vi "L12_1.1.vi"() -> ()   [LabVIEW 2012]
panel:
  out "sum":i64
  out "max index(es)":i32
  out "max value":dbl
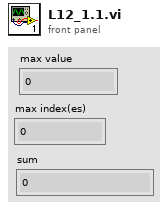
[diagram p1: front panel]
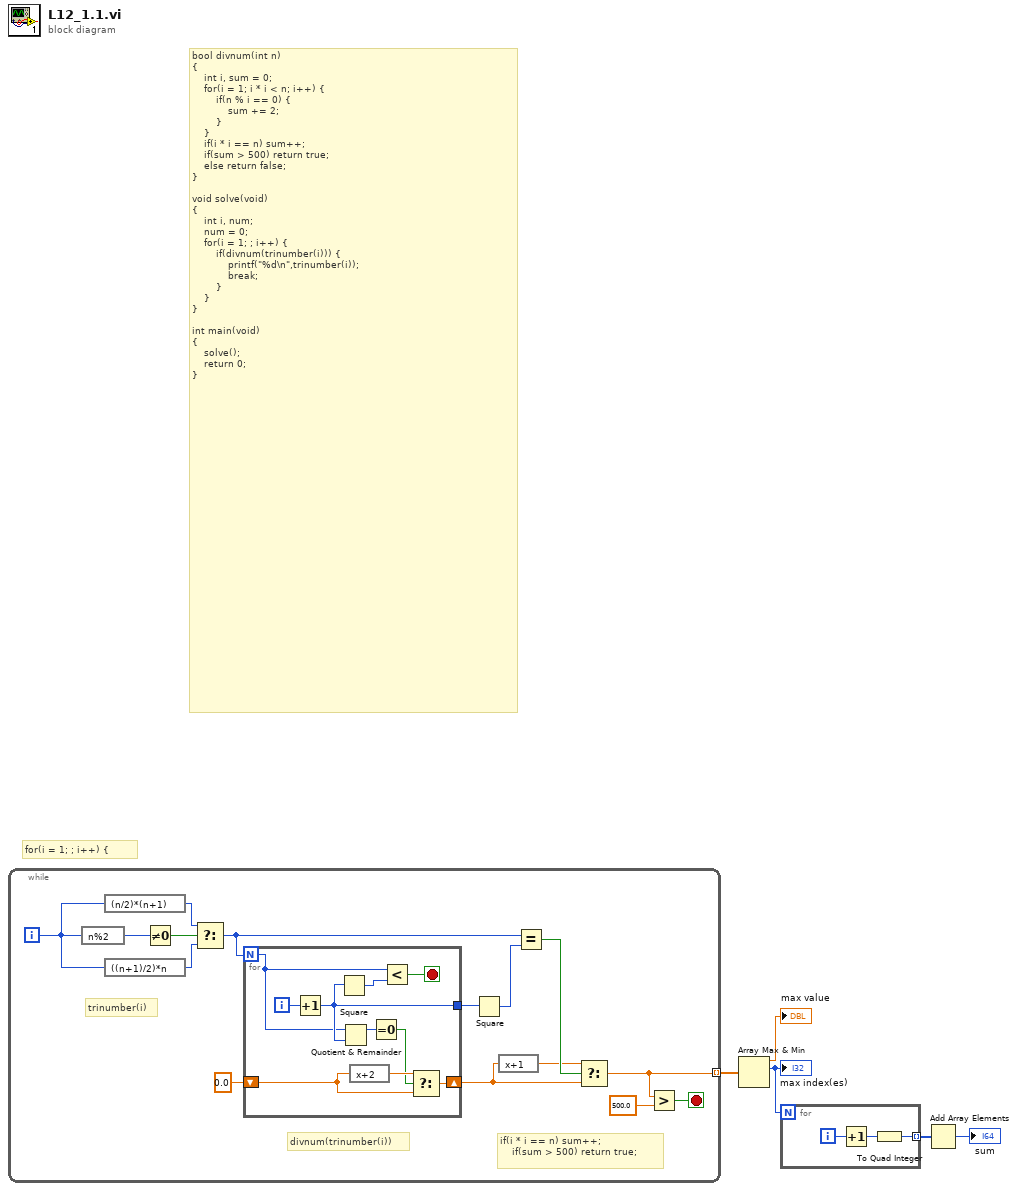
[diagram p0: block diagram]
diagram:
  # "for(i = 1; ; i++) {"
  # "bool divnum(int n)  \n{  \n    int i, sum = 0;  \n    for(i = 1; i * i < n; i++) {  \n        if(n % i == 0) {  \n            sum += 2;  \n        }  \n    }  \n    if(i * i == n) sum++;  \n    if(sum > 500) return true;  \n    else return false;  \n}  \n  \nvoid solve(void)  \n{  \n    int i, num;  \n    num = 0;  \n    for(i = 1; ; i++) {  \n        if(divnum(trinumber(i))) {  \n            printf(\"%d\\n\",trinumber(i));  \n            break;  \n        }  \n    }  \n}  \n  \nint main(void)  \n{  \n    solve();  \n    return 0;  \n}"
  n1 = while {
    tunnel: [w9] -> w5 mode=indexing
    i -> [w7]
    stop <- w6 stop-if-true
    # "if(i * i == n) sum++;  \n    if(sum > 500) return true;"
    # "divnum(trinumber(i))"
    # "trinumber(i)"
    n2 = expression code="n%2"(w7) -> (w20:i32)
    n3 = expression code="(n/2)*(n+1)"(w7) -> (w18:i32)
    n4 = expression code="((n+1)/2)*n"(w7) -> (w17:i32)
    n5 = Not Equal To 0?(x=w20) -> (x != 0?=w19:bool)
    n6 = Select(t=w18, s=w19, f=w17) -> (s? t:f=w13:i32)
    n7 = for {
      N: w13 -> [w21]
      shift-right: [w26] -> w10
      shift-left: 0.0 -> [w24]
      tunnel: [w28] -> w15
      i -> [w30]
      stop <- w29 stop-if-true
      n8 = Increment(x=w30) -> (x+1=w28:i32)
      n9 = Square(x=w28) -> (x^2=w22:i32)
      n10 = Quotient & Remainder(x=w21, y=w28) -> (x-y*floor(x/y)=w27:i32)  [unwired: 1 out]
      n11 = expression code="x+2"(w24) -> (w25:dbl)
      n12 = Equal To 0?(x=w27) -> (x = 0?=w23:bool)
      n13 = Less?(x=w21, y=w22) -> (x < y?=w29:bool)
      n14 = Select(t=w25, s=w23, f=w24) -> (s? t:f=w26:dbl)
    }
    n15 = Square(x=w15) -> (x^2=w14:i32)
    n16 = expression code="x+1"(w10) -> (w11:dbl)
    n17 = Equal?(x=w13, y=w14) -> (x = y?=w12:bool)
    n18 = Select(t=w11, s=w12, f=w10) -> (s? t:f=w9:dbl)
    n19 = Greater?(x=w9, y=500.0) -> (0:w6:bool)
  }
  n20 = Array Max & Min(array=w5) -> (max value=→"max value":dbl, max index (indices)=w3:i32)  [unwired: 2 out]
  "max index(es)" <- w3
  n21 = for {
    N: w3 -> [_]
    tunnel: [w32] -> w2 mode=indexing
    i -> [w33]
    n22 = Increment(x=w33) -> (x+1=w31:i32)
    n23 = To Quad Integer(1:w31) -> (0:w32:i64)
  }
  n24 = Add Array Elements(numeric array=w2) -> (sum=→"sum":i64)
